vi "add tag with retry.vi"(5 "retrys allowed":i32=20, 7 "owner ID":string, 8 "error in":errorcluster, 10 "tag in":refnum<class "tag descriptor.lvclass">, 11 "engine configuration in":refnum<class "engine configuration.lvclass">) -> (0 "error out":errorcluster, 2 "tag out":refnum<class "tag descriptor.lvclass">, 3 "engine configuration out":refnum<class "engine configuration.lvclass">)   [LabVIEW 2013, in "engine configuration.lvclass"]
uses:
  engine configuration.lvclass
  <vilib>/NI/Tag Bus/tag/tag descriptor.lvclass
  <vilib>/NI/Tag Bus/tag/tag descriptor.lvclass/tag descriptor.ctl
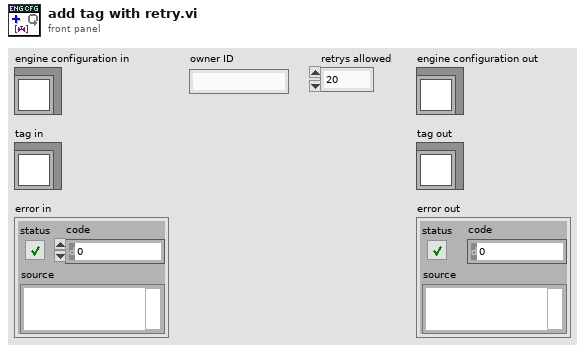
[diagram p1: front panel]
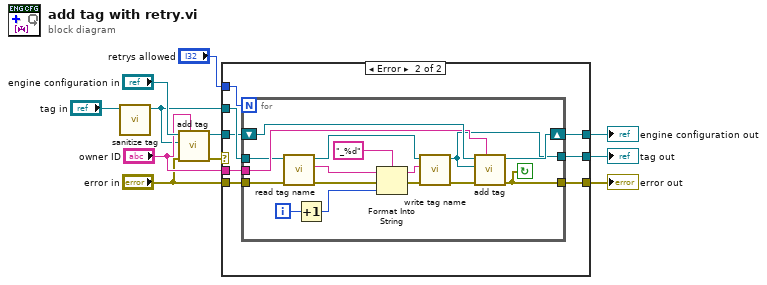
[diagram p0: block diagram]
diagram:
  n1 = call "sanitize tag.vi"("tag descriptor"="tag in") -> ("clean tag"=w1:refnum<class "tag descriptor.lvclass">)  [unwired: 10 in]
  n2 = call-dynamic "add tag.vi"("owner ID"="owner ID", "error in"="error in", "tag descriptor"=w1, "engine configuration in"="engine configuration in") -> ("error out"=w3:errorcluster, "engine configuration out"=w5:refnum<class "engine configuration.lvclass">)  [unwired: 6 in]
  n3 = case shown="Error" w3 {
    selector: w3 -> [w14 _]
    tunnel: [w13 w22] -> w11
    tunnel: [w12 w21] -> w10
    tunnel: [w14 w20] -> w9
    tunnel: "retrys allowed" -> [_ w19]
    tunnel: w1 -> [w13 w18]
    tunnel: w5 -> [w12 w17]
    tunnel: "owner ID" -> [_ w16]
    tunnel: "error in" -> [_ w15]
    frame No Error {
    }
    frame Error {
      n4 = for {
        N: w19 -> [_]
        shift-right: [w38] -> w21
        shift-left: w17 -> [w37]
        tunnel: w15 -> [w36]
        tunnel: w18 -> [w32]
        tunnel: [w29] -> w22
        tunnel: [w35] -> w20
        tunnel: w16 -> [w34]
        i -> [w25]
        stop <- w35 continue-if-true
        n5 = call <vilib>:"read tag name.vi"("error in"=w36, "system tag in"=w32) -> ("error out"=w33:errorcluster, "name"=w26:string, "system tag out"=w30:refnum<class "tag descriptor.lvclass">)  [unwired: 7 in]
        n6 = Increment(x=w25) -> (x+1=w23:i32)
        n7 = Format Into String(format string="_%d", initial string=w26, error in=w33, w23) -> (resulting string=w27:string, error out=w28:errorcluster)
        n8 = call <vilib>:"write tag name.vi"("error in"=w28, "name"=w27, "system tag in"=w30) -> ("error out"=w31:errorcluster, "system tag out"=w29:refnum<class "tag descriptor.lvclass">)  [unwired: 7 in]
        n9 = call-dynamic "add tag.vi"("owner ID"=w34, "error in"=w31, "tag descriptor"=w29, "engine configuration in"=w37) -> ("error out"=w35:errorcluster, "engine configuration out"=w38:refnum<class "engine configuration.lvclass">)  [unwired: 6 in]
      }
    }
  }
  "tag out" <- w11
  "engine configuration out" <- w10
  "error out" <- w9
